vi "KeyenceCVX.Main.StatusUpdate.vi"(8 "error in":errorcluster, 11 "Data in":T1) -> (0 "error out":errorcluster)   [LabVIEW 2016]
uses:
  KeyenceCVX.Data.ctl
  KeyenceCVX.Data.Status.ctl
  KeyenceCVX.Data.Status.State.ctl
  KeyenceCVX.Data.Sets.ctl
  KeyenceCVX.CodeDetails.ctl
  Keyence/LowLevel/Keyence.Global.vi
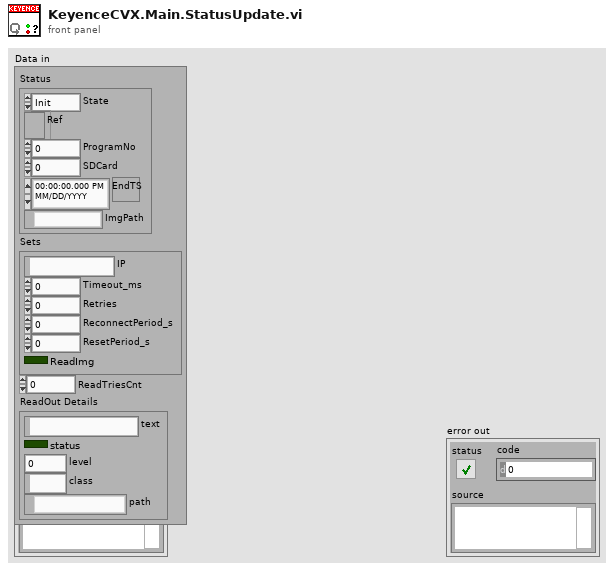
[diagram p1: front panel]
types:
  T1 = typedef "KeyenceCVX.Data.ctl" = cluster{"Status":T2, "Sets":T4, "ReadTriesCnt":u8, "ReadOut Details":T5}
  T2 = typedef "KeyenceCVX.Data.Status.ctl" = cluster{"State":T3, "Ref":refnum<k5>, "ProgramNo":u16, "SDCard":u8, "EndTS":timestamp, "ImgPath":path}
  T3 = typedef "KeyenceCVX.Data.Status.State.ctl" = enum16{"Init", "Reset", "Idle", "Scan"}
  T4 = typedef "KeyenceCVX.Data.Sets.ctl" = cluster{"IP":string, "Timeout_ms":i32, "Retries":i32, "ReconnectPeriod_s":i32, "ResetPeriod_s":i32, "ReadImg":bool}
  T5 = typedef "KeyenceCVX.CodeDetails.ctl" = cluster{"text":string, "status":bool, "level":u8, "class":string, "path":path}
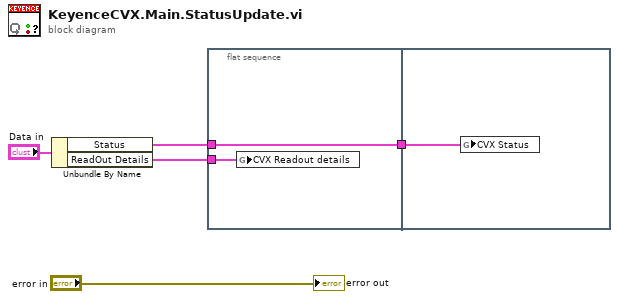
[diagram p0: block diagram]
diagram:
  n1 = Unbundle By Name("Data in") -> ("Status"=w4:T2, "ReadOut Details"=w3:T5)
  n2 = flat-sequence {
    tunnel: w4 -> [w6]
    tunnel: w3 -> [w7]
    tunnel: [w6] -> w2
    tunnel: w2 -> [w8]
    frame #0 {
      n3 = global write "Keyence.Global.vi" "CVX Readout details"(w7) -> ()
    }
    frame #1 {
      n4 = global write "Keyence.Global.vi" "CVX Status"(w8) -> ()
    }
  }
  "error out" <- "error in"
